vi "Initialize (VISA).vi"(7 "Force Baud Rate (True)":bool=TRUE, 8 "error in (no error)":errorcluster, 9 "Timeout (30 msec)":u32=30, 10 "Baud rate (57600 bps)":T1=34 items=["1,000,000 bps"=1, "500,000 bps"=3, "400,000 bps"=4, "250,000 bps"=7, "200,000 bps"=9, "115200 bps"=16, "57600 bps"=34, "19200 bps"=103, "9600 bps"=207], 11 "VISA resource name":refnum<visa-resource-name>) -> (0 "error out":errorcluster, 3 "Dynamixel Motor out":refnum<class "Dynamixel Motor.lvclass">)   [LabVIEW 2016, in "Dynamixel Motor VISA.lvclass"]
doc: "Establishes communication with the sensor. It also places the sensor in a default state needed for other sensor driver operations. Therefore, call this VI before calling other sensor driver VIs for this sensor. Generally, you need to call the Initialize VI only once at the beginning of an application."
uses:
  <instrlib>/Dynamixel Motor/HAIOL/VISA/Dynamixel Motor VISA.lvclass
  <instrlib>/Dynamixel Motor/Public/Motor Operation/Low Level/Baud Setting.ctl
  <instrlib>/Dynamixel Motor/HAIOL/Dynamixel Motor.lvclass
  c:/Program Files (x86)/National Instruments/LabVIEW 2016/instr.lib/Dynamixel Motor/HAIOL/Dynamixel Motor.lvclass
  <instrlib>/Dynamixel Motor/HAIOL/VISA/Dynamixel Motor VISA.lvclass/Dynamixel Motor VISA.ctl
  <instrlib>/Dynamixel Motor/Dynamixel Motor.lvlib
panel:
  # "(c) 2011  National Instruments.  ALL RIGHTS RESERVED."
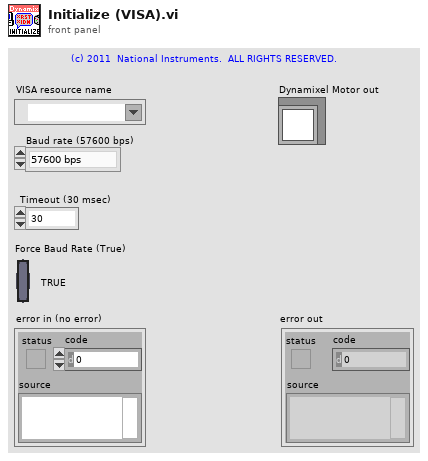
[diagram p1: front panel]
types:
  T1 = typedef "Dynamixel Motor.lvlib/Baud Setting.ctl" = u8
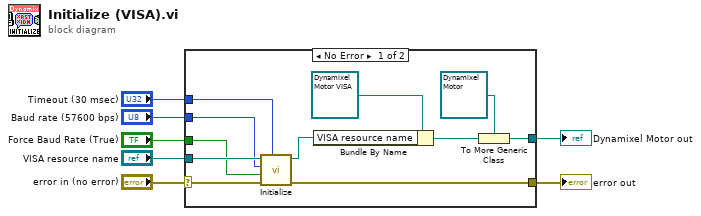
[diagram p0: block diagram]
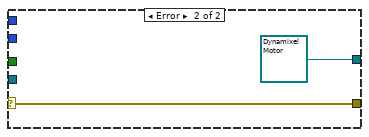
[diagram p2: hidden frame]
diagram:
  n1 = case shown="No Error" "error in (no error)" {
    selector: "error in (no error)" -> [w18 w19]
    tunnel: "VISA resource name" -> [w17 _]
    tunnel: "Baud rate (57600 bps)" -> [w16 _]
    tunnel: "Force Baud Rate (True)" -> [w15 _]
    tunnel: "Timeout (30 msec)" -> [w14 _]
    tunnel: [w13 w19] -> w1
    tunnel: [w8 refnum<class "Dynamixel Motor.lvclass"> refnum ("Dynamixel Motor.lvclass")] -> w2
    frame No Error {
      n2 = call <instrlib>:"Initialize.vi"("Timeout (30 msec)"=w14, "error in (no error)"=w18, "Force Baud Rate (True)"=w15, "Baud rate (57600 bps)"=w16, "VISA resource name"=w17) -> ("error out"=w13:errorcluster, "VISA resource name out"=w12:refnum<visa-resource-name>)  [unwired: 5 in]
      n3 = Bundle By Name(cluster=refnum<class "Dynamixel Motor VISA.lvclass"> refnum ("Dynamixel Motor VISA.lvclass"), "VISA resource name"=w12) -> (w10:refnum<class "Dynamixel Motor VISA.lvclass">)
      n4 = To More Generic Class(target class=refnum<class "Dynamixel Motor.lvclass"> refnum ("Dynamixel Motor.lvclass"), reference=w10) -> (generic class reference=w8:refnum<class "Dynamixel Motor.lvclass">)
    }
    frame Error {
    }
  }
  "error out" <- w1
  "Dynamixel Motor out" <- w2
